vi "svx_Colormap Facade.vi"(0 "Data In":T5 {"Y scale"."multiplier" format="%.2f"; "Y scale"."offset" format="%.2f"; "X scale"."multiplier" format="%.2f"; "X scale"."offset" format="%.2f"; "spectral map" format="%.2f"}, 2 "Display State In":T3={"RefQueue"=refnum, "Properties/Undo"=refnum, "Bound"={"Width"=0, "Height"=0}, "Plot Area:Colors"={"FG Color"=11776947, "BG Color"=0}, "scale legend visible?"=FALSE, "graph palette visible?"=FALSE, "cursor palette visible?"=FALSE, "Ignore Array"=TRUE, "Smooth Update"=FALSE, "Z Scale"={"Z Scale.Scale Fit"=2, "Z Scale.Name Label.Text"="Amplitude", "Z Scale.Interpolate Color"=TRUE, "Visible"=TRUE, "Label Visible"=TRUE, "format string"="%#.2g", "Z Scale.Range"={"Minimum"=0.0, "Maximum"=500.0}}, "X Scale"={"X Scale.Scale Fit"=2, "X Scale.Offset and Multiplier"={"Offset"=0.0, "Multiplier"=1.0}, "X Scale.Name Label.Text"="Time", "X Scale.Range"={"Minimum"=0.0, "Maximum"=10.0}, "Visible"=TRUE, "Label Visible"=TRUE, "format string"="%#.2g"}, "Y Scale"={"Y Scale.Scale Fit"=2, "Y Scale.Offset and Multiplier"={"Offset"=0.0, "Multiplier"=1.0}, "Y Scale.Name Label.Text"="Frequency", "Y Scale.Range"={"Minimum"=0.0, "Maximum"=500.0}, "Visible"=TRUE, "Label Visible"=TRUE, "format string"="%#.2g"}, "Annotation List"=[], "Cursor List"=[], "Display Frequency Lines"=TRUE, "Display Order Lines"=TRUE, "Display Order text"=TRUE, "Display Frequency text"=TRUE, "Order Lineproperty"={"Line"={"Width"=1, "Style"=enum."Dash"}, "color"=0}, "Order Textproperty"={"Test size"=11, "color"=16777222, "background"=16777216}, "Orders"=[], "Frequency"=[], "Frequency Lineproperty"={"Line"={"Width"=1, "Style"=enum."Dash"}, "color"=0}, "Frequency Textproperty"={"Test size"=11, "color"=16777222, "background"=16777216}, "Display Order from Cursor"=FALSE, "Display Freq from Cursor"=FALSE, "Active Cursor"=0, "Selected Cursors"=[], "Cursor Move"=refnum, "Scale Range Change"=refnum}, 3 "Container State":T4) -> (6 "Data Out":T5 {"Y scale"."multiplier" format="%.2f"; "Y scale"."offset" format="%.2f"; "X scale"."multiplier" format="%.2f"; "X scale"."offset" format="%.2f"; "spectral map" format="%.2f"}, 7 "Display State Out":T3={"RefQueue"=refnum, "Properties/Undo"=refnum, "Bound"={"Width"=0, "Height"=0}, "Plot Area:Colors"={"FG Color"=11776947, "BG Color"=0}, "scale legend visible?"=FALSE, "graph palette visible?"=FALSE, "cursor palette visible?"=FALSE, "Ignore Array"=TRUE, "Smooth Update"=FALSE, "Z Scale"={"Z Scale.Scale Fit"=2, "Z Scale.Name Label.Text"="Amplitude", "Z Scale.Interpolate Color"=TRUE, "Visible"=TRUE, "Label Visible"=TRUE, "format string"="%#.2g", "Z Scale.Range"={"Minimum"=0.0, "Maximum"=500.0}}, "X Scale"={"X Scale.Scale Fit"=2, "X Scale.Offset and Multiplier"={"Offset"=0.0, "Multiplier"=1.0}, "X Scale.Name Label.Text"="Time", "X Scale.Range"={"Minimum"=0.0, "Maximum"=10.0}, "Visible"=TRUE, "Label Visible"=TRUE, "format string"="%#.2g"}, "Y Scale"={"Y Scale.Scale Fit"=2, "Y Scale.Offset and Multiplier"={"Offset"=0.0, "Multiplier"=1.0}, "Y Scale.Name Label.Text"="Frequency", "Y Scale.Range"={"Minimum"=0.0, "Maximum"=500.0}, "Visible"=TRUE, "Label Visible"=TRUE, "format string"="%#.2g"}, "Annotation List"=[], "Cursor List"=[], "Display Frequency Lines"=TRUE, "Display Order Lines"=TRUE, "Display Order text"=TRUE, "Display Frequency text"=TRUE, "Order Lineproperty"={"Line"={"Width"=1, "Style"=enum."Dash"}, "color"=0}, "Order Textproperty"={"Test size"=11, "color"=16777222, "background"=16777216}, "Orders"=[], "Frequency"=[], "Frequency Lineproperty"={"Line"={"Width"=1, "Style"=enum."Dash"}, "color"=0}, "Frequency Textproperty"={"Test size"=11, "color"=16777222, "background"=16777216}, "Display Order from Cursor"=FALSE, "Display Freq from Cursor"=FALSE, "Active Cursor"=0, "Selected Cursors"=[], "Cursor Move"=refnum, "Scale Range Change"=refnum}, 8 "Action":T2)   [LabVIEW 2017, in "SVX Colormap.xctl"]
uses:
  <vilib>/addons/_XControls/Colormap/SVX Colormap.xctl
  <vilib>/addons/_XControls/Colormap/subVIs/svx_Colormap Data.ctl
  <vilib>/_xctls/Container State.ctl
  <vilib>/addons/_XControls/Colormap/subVIs/svx_Colormap State.ctl
  <vilib>/addons/_XControls/Colormap/TypeDef/svx_Colormap_InnerState.ctl
  <vilib>/addons/_XControls/Colormap/TypeDef/svx_Colormap_Event.ctl
  <vilib>/_xctls/Action.ctl
  <vilib>/Utility/miscctls.llb/LVPoint32TypeDef.ctl
  <vilib>/_xctls/XControlSupport.lvlib
panel:
  in  "by cursor legend?":bool=TRUE
  out "Coords":T1
  out "Colormap":dbl[][](graph)
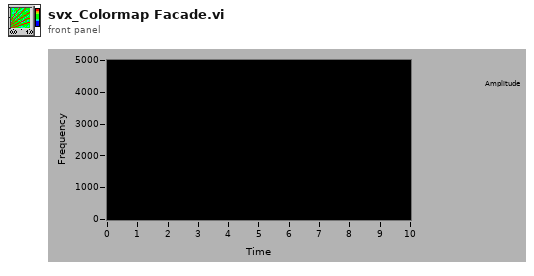
[diagram p1: front panel]
types:
  T1 = typedef "LVPoint32TypeDef.ctl" = cluster{"Horizontal":i32, "Vertical":i32}
  T2 = typedef "XControlSupport.lvlib/Action.ctl" = cluster{"Data Changed?":bool, "State Changed?":bool, "Action Name":string}
  T3 = typedef "SVX Colormap.xctl/svx_Colormap State.ctl" = cluster{"RefQueue":refnum<queue>, "Properties/Undo":refnum<queue>, "Bound":cluster{"Width":u32, "Height":u32}, "Plot Area:Colors":cluster{"FG Color":u32, "BG Color":u32}, "scale legend visible?":bool, "graph palette visible?":bool, "cursor palette visible?":bool, "Ignore Array":bool, "Smooth Update":bool, "Z Scale":cluster{"Z Scale.Scale Fit":u8, "Z Scale.Name Label.Text":string, "Z Scale.Interpolate Color":bool, "Visible":bool, "Label Visible":bool, "format string":string, "Z Scale.Range":cluster{"Minimum":dbl, "Maximum":dbl}}, "X Scale":cluster{"X Scale.Scale Fit":u8, "X Scale.Offset and Multiplier":cluster{"Offset":dbl, "Multiplier":dbl}, "X Scale.Name Label.Text":string, "X Scale.Range":cluster{"Minimum":dbl, "Maximum":dbl}, "Visible":bool, "Label Visible":bool, "format string":string}, "Y Scale":cluster{"Y Scale.Scale Fit":u8, "Y Scale.Offset and Multiplier":cluster{"Offset":dbl, "Multiplier":dbl}, "Y Scale.Name Label.Text":string, "Y Scale.Range":cluster{"Minimum":dbl, "Maximum":dbl}, "Visible":bool, "Label Visible":bool, "format string":string}, "Annotation List":cluster{"Name":string, "Color":u32, "Style":u8, "Point Style":u8, "Name Visible":bool, "Allow Drag":bool, "Annotation Mode":u32, "Plot":i32, "Index":i32, "Position":cluster{"X":dbl, "Y":dbl}, "X Scale":u32, "Y Scale":u32, "Show Arrow":bool, "Lock Name":bool, "Plot Area":i32, "Label Offset":cluster{"X":dbl, "Y":dbl}}[], "Cursor List":cluster{"Name":string, "Color":u32, "Style":u8, "Point Style":u8, "Name Visible":bool, "Allow Drag":bool, "Cursor Mode":u32, "Plot":i32, "Index":i32, "Position":cluster{"X":dbl, "Y":dbl}, "X Scale":u32, "Y Scale":u32, "Watch Plots":i32[], "Watch All Plots":bool, "Plot Area":i32, "Label Offset":cluster{"X":dbl, "Y":dbl}}[], "Display Frequency Lines":bool, "Display Order Lines":bool, "Display Order text":bool, "Display Frequency text":bool, "Order Lineproperty":cluster{"Line":cluster{"Width":u16, "Style":enum32{"Solid", "Dash", "Dot", "DashDot", "DashDotDot"}}, "color":u32}, "Order Textproperty":cluster{"Test size":i16, "color":u32, "background":u32}, "Orders":dbl[], "Frequency":dbl[], "Frequency Lineproperty":cluster{"Line":cluster{"Width":u16, "Style":enum32{"Solid", "Dash", "Dot", "DashDot", "DashDotDot"}}, "color":u32}, "Frequency Textproperty":cluster{"Test size":i16, "color":u32, "background":u32}, "Display Order from Cursor":bool, "Display Freq from Cursor":bool, "Active Cursor":u32, "Selected Cursors":u32[], "Cursor Move":refnum<user-event>, "Scale Range Change":refnum<user-event>}
  T4 = typedef "XControlSupport.lvlib/Container State.ctl" = cluster{"Indicator?":bool, "Run Mode?":bool, " Refnum":refnum<vi>}
  T5 = typedef "SVX Colormap.xctl/svx_Colormap Data.ctl" = cluster{"spectral map":dbl[][], "X scale":cluster{"offset":dbl, "multiplier":dbl}, "Y scale":cluster{"offset":dbl, "multiplier":dbl}, "attribute":variant}
  T6 = cluster{"Minimum":dbl, "Maximum":dbl, "Kind":enum16{"X-Scale", "Y-Scale", "Z-Scale"}}
  T7 = typedef "SVX Colormap.xctl/svx_Colormap_Event.ctl" = enum16{"None", "[Axis] X Range", "[Axis] Y Range", "[Axis] Z Range", "[Axis] Range", "[Axis] X FString", "[Axis] Y FString", "[Axis] Z FString", "[Axis] X Name", "[Axis] X ScaleVis", "[Axis] X NameVis", "[Axis] Y Name", "[Axis] Y ScaleVis", "[Axis] Y NameVis", "[Axis] Z Name", "[Axis] Z ScaleVis", "[Axis] Z NameVis", "[Image] Line", "[Axis] Z Interp", "[Data] Update", "[Layout] Resize", "[ColorTable] Ignore Array", "[Legend] ScaleVis", "[Legend] GPVis", "[Legend] CPVis", "[Smooth] Update", "[Cursor] Update", "[Plot Area] Colors", "[Size] Minimum", "[Annotation] Update", "[Properties Dialog]", "[Axis] Autoscale X", "[Axis] Autoscale Y", "[Axis] Autoscale Z"}
  T8 = typedef "LVRectTypeDef.ctl" = cluster{"Left":i16, "Top":i16, "Right":i16, "Bottom":i16}
  T9 = typedef "LVCursorListTypeDef.ctl" = cluster{"Name":string, "Color":u32, "Style":u8, "Point Style":u8, "Name Visible":bool, "Allow Drag":bool, "Cursor Mode":u32, "Plot":i32, "Index":i32, "Position":cluster{"X":dbl, "Y":dbl}, "X Scale":u32, "Y Scale":u32, "Watch Plots":i32[], "Watch All Plots":bool, "Plot Area":i32, "Label Offset":cluster{"X":dbl, "Y":dbl}}[]
  T10 = cluster{"Shift":bool, "Ctrl":bool, "Alt":bool, "Cmd":bool, "Opt":bool}
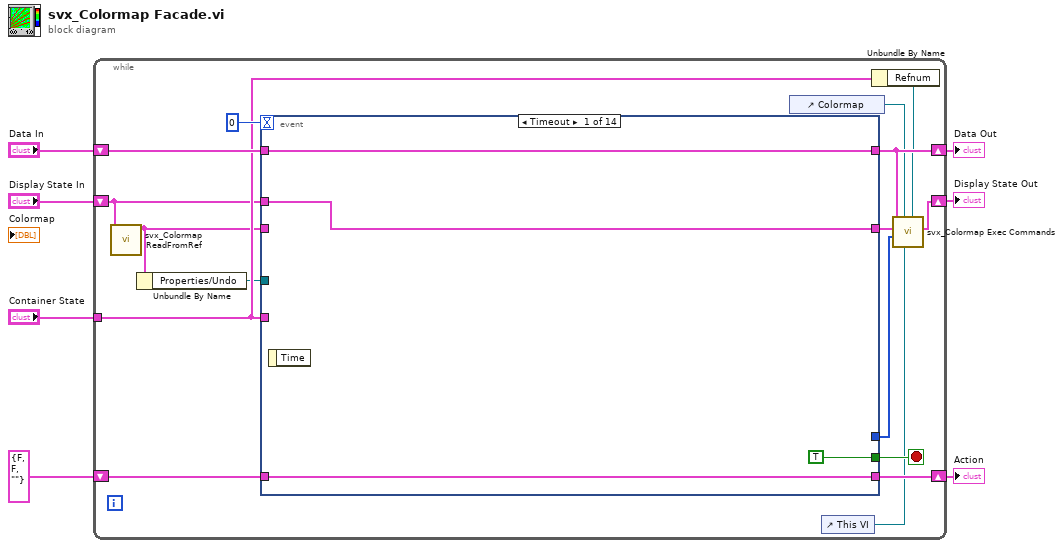
[diagram p0: block diagram]
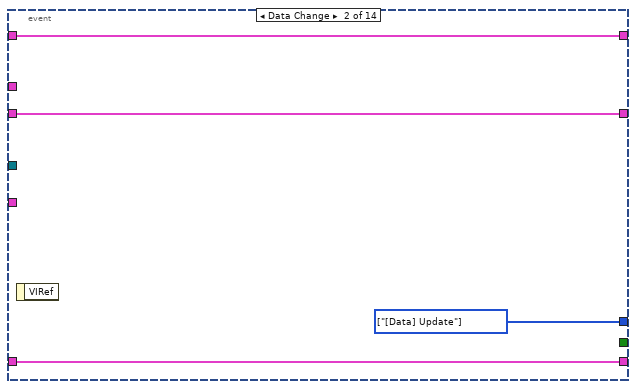
[diagram p2: hidden frame]
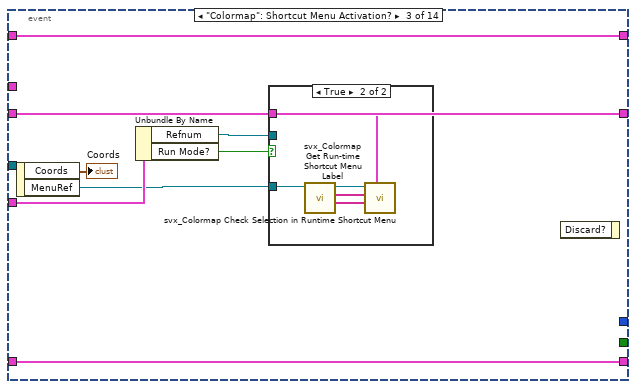
[diagram p3: hidden frame]
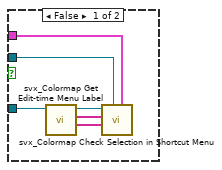
[diagram p4: hidden frame]
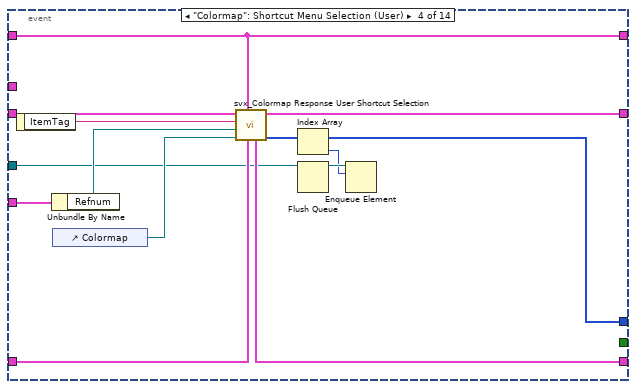
[diagram p5: hidden frame]
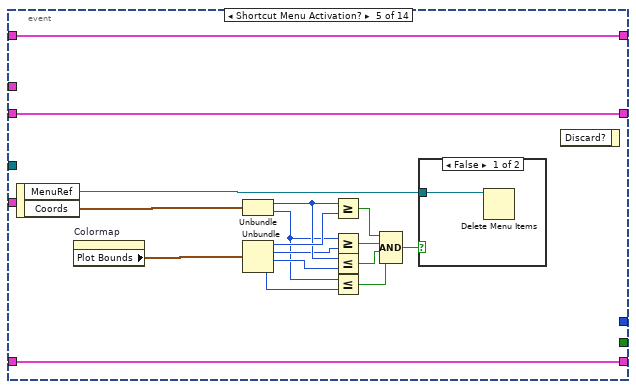
[diagram p6: hidden frame]
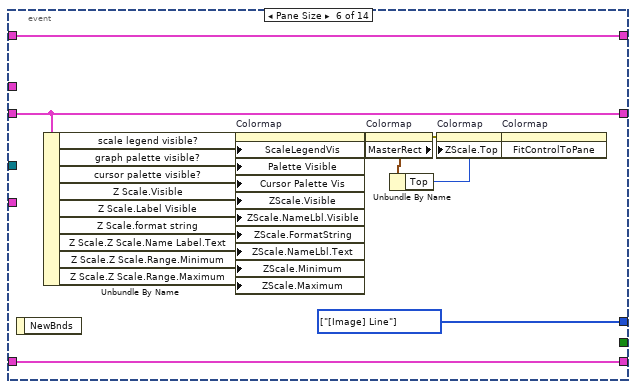
[diagram p8: hidden frame]
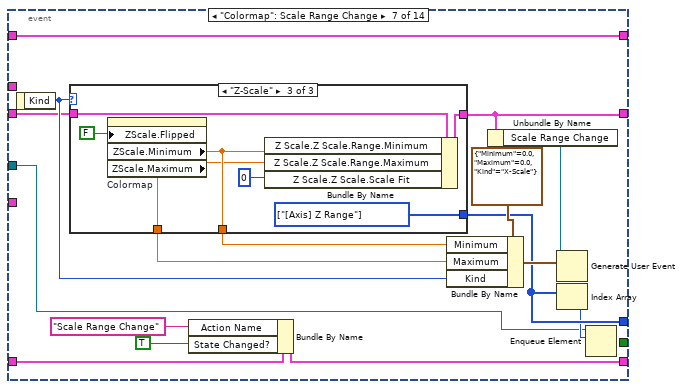
[diagram p9: hidden frame]
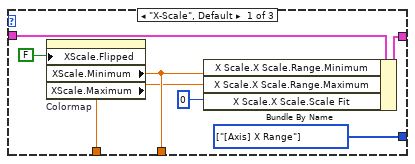
[diagram p10: hidden frame]
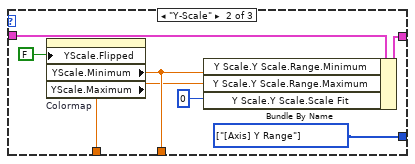
[diagram p11: hidden frame]
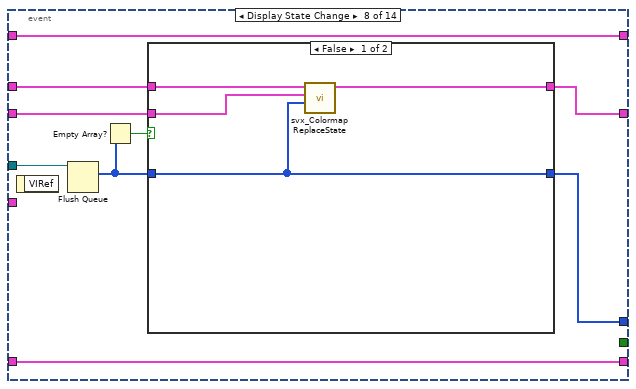
[diagram p12: hidden frame]
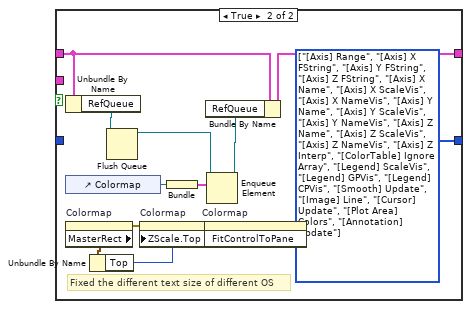
[diagram p13: hidden frame]
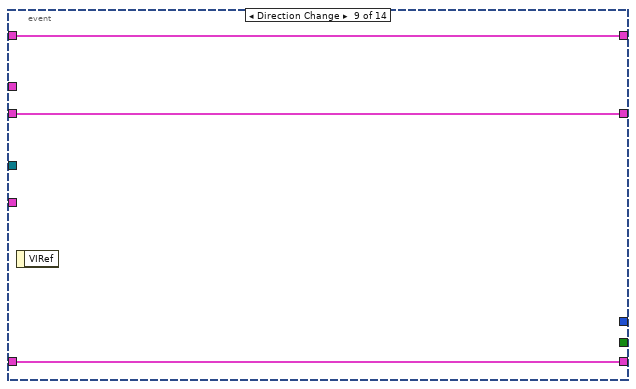
[diagram p14: hidden frame]
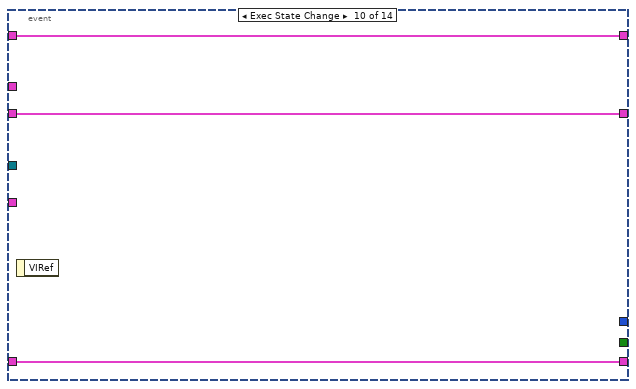
[diagram p15: hidden frame]
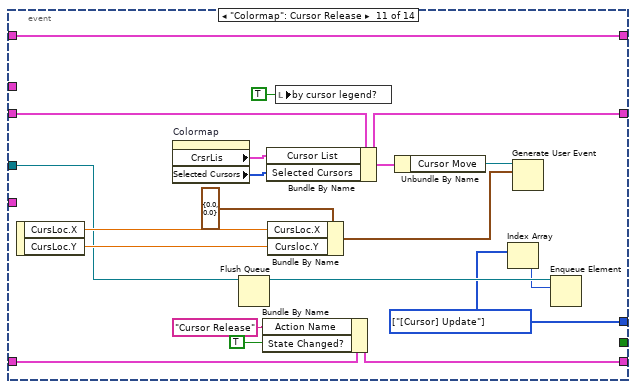
[diagram p16: hidden frame]
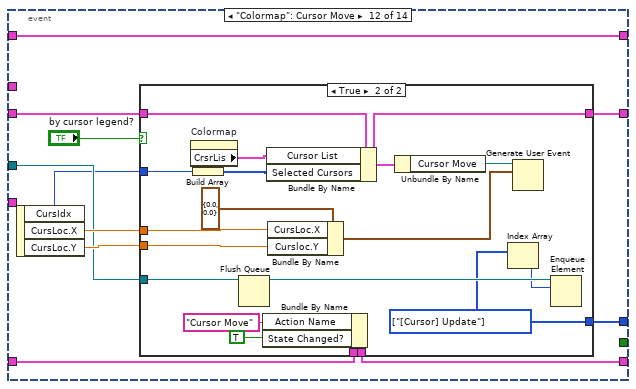
[diagram p17: hidden frame]
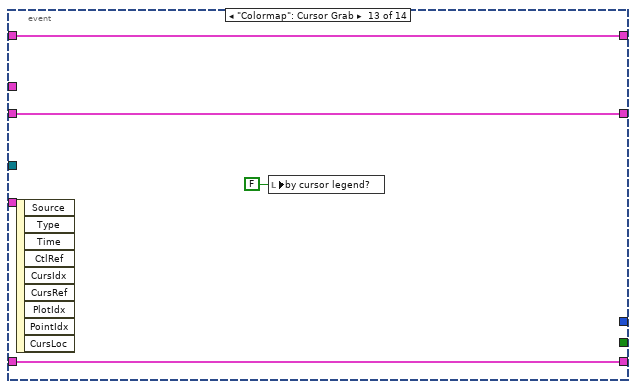
[diagram p19: hidden frame]
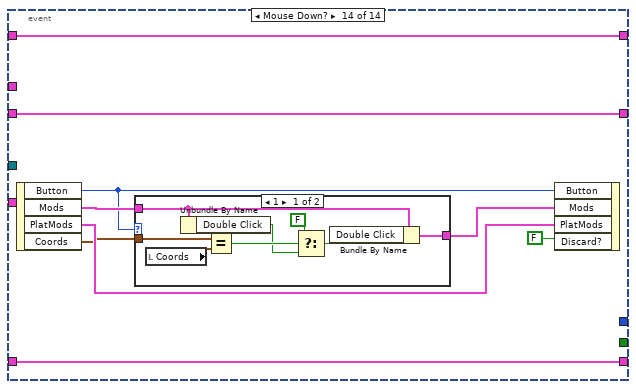
[diagram p20: hidden frame]
diagram:
  n1 = while {
    shift-right: [w8] -> w4
    shift-left: "Display State In" -> [w10]
    tunnel: "Container State" -> [w19]
    shift-right: [w20] -> w2
    shift-left: "Data In" -> [w22]
    shift-right: [w15] -> w3
    shift-left: T2 {"Data Changed?"=FALSE, "State Changed?"=FALSE, "Action Name"=""} ("Action") -> [w21]
    stop <- w13 stop-if-true
    n2 = call <vilib>:"svx_Colormap ReadFromRef.vi"("State in"=w10) -> ("State out"=w11:T3)  [unwired: 10 in]
    n3 = Unbundle By Name(w11) -> ("Properties/Undo"=w14:refnum<queue>)
    n4 = event shown="[0] Timeout" {
      selector: _ -> [_ _ _ _ _ _ _ _ _ _ _ _ _ _]
      dyn-events: _ -> [_ _ _ _ _ _ _ _ _ _ _ _ _ _]
      timeout: 0 -> [_ _ _ _ _ _ _ _ _ _ _ _ _ _]
      tunnel: w19 -> [_ _ w36 w61 _ _ _ _ _ _ _ _ _ _]
      tunnel: w22 -> [w27 w31 w39 w60 w79 w98 w111 w145 w164 w167 w183 w195 w219 w230]
      tunnel: [w27 w31 w39 w60 w79 w98 w111 w145 w164 w167 w183 w195 w219 w230] -> w20
      tunnel: [w26 w30 w38 w62 w80 w99 w113 w144 w163 w166 w184 w196 w218 w228] -> w15
      tunnel: w21 -> [w26 w30 w38 w63 w80 w99 w114 w144 w163 w166 w185 w197 w218 w228]
      tunnel: w10 -> [w24 _ _ _ _ _ _ w139 _ _ _ _ _ _]
      tunnel: w14 -> [_ _ _ w52 _ _ w100 w143 _ _ w172 w190 _ _]
      tunnel: [_ w29 _ w51 _ w97 w102 w140 _ _ w170 w189 _ _] -> w16
      tunnel: w11 -> [_ w28 w33 w59 w64 w82 w105 w137 w162 w165 w177 w192 w220 w229]
      tunnel: [w24 w28 w33 w58 w64 w82 w104 w138 w162 w165 w175 w191 w220 w229] -> w9
      tunnel: [TRUE _ _ _ _ _ _ _ _ _ _ _ _ _] -> w13
      event Timeout {
        n5 = event-data() -> ()  [unwired: 1 in, 1 out]
      }
      event Data Change {
        w29 = T7[] [enum."[Data] Update"] items=["None", "[Axis] X Range", "[Axis] Y Range", "[Axis] Z Range", "[Axis] Range", "[Axis] X FString", "[Axis] Y FString", "[Axis] Z FString", "[Axis] X Name", "[Axis] X ScaleVis", "[Axis] X NameVis", "[Axis] Y Name", "[Axis] Y ScaleVis", "[Axis] Y NameVis", "[Axis] Z Name", "[Axis] Z ScaleVis", "[Axis] Z NameVis", "[Image] Line", "[Axis] Z Interp", "[Data] Update", "[Layout] Resize", "[ColorTable] Ignore Array", "[Legend] ScaleVis", "[Legend] GPVis", "[Legend] CPVis", "[Smooth] Update", "[Cursor] Update", "[Plot Area] Colors", "[Size] Minimum", "[Annotation] Update", "[Properties Dialog]", "[Axis] Autoscale X", "[Axis] Autoscale Y", "[Axis] Autoscale Z"]
        n6 = event-data() -> ()  [unwired: 1 in, 1 out]
      }
      event "Colormap": Shortcut Menu Activation? {
        n7 = event-data() -> ("Coords"=→"Coords":T1, "MenuRef"=w34:refnum<k9>)  [unwired: 1 in]
        n8 = Unbundle By Name(w36) -> ("Refnum"=w35:refnum<vi>, "Run Mode?"=w37:bool)
        n9 = case shown="True" w37 {
          tunnel: w34 -> [w45 w50]
          tunnel: w35 -> [w42 _]
          tunnel: w33 -> [w41 w46]
          frame False {
            n10 = call <vilib>:"svx_Colormap Get Edit-time Menu Label.vi"("MenuRef"=w45) -> ("Disable item tags"=w40:string[], "item tags"=w43:string[], "menu reference out"=w44:refnum<k9>)  [unwired: 8 in]
            n11 = call <vilib>:"svx_Colormap Check Selection in Shortcut Menu.vi"("State"=w41, "Refnum"=w42, "Disable item tags"=w40, "item tags"=w43, "menu reference in"=w44) -> ()  [unwired: 7 in]
          }
          frame True {
            n12 = call <vilib>:"svx_Colormap Get Run-time Shortcut Menu Label.vi"("MenuRef"=w50) -> ("Disable item tags"=w47:string[], "item tags"=w48:string[], "menu reference out"=w49:refnum<k9>)  [unwired: 8 in]
            n13 = call <vilib>:"svx_Colormap Check Selection in Runtime Shortcut Menu.vi"("State"=w46, "Disable item tags"=w47, "item tags"=w48, "menu reference in"=w49) -> ()  [unwired: 8 in]
          }
        }
        n14 = event-data() -> ()  [unwired: 2 in, 1 out]
      }
      event "Colormap": Shortcut Menu Selection (User) {
        n15 = event-data() -> ("ItemTag"=w57:string)  [unwired: 1 in]
        n16 = Unbundle By Name(w61) -> ("Refnum"=w56:refnum<vi>)
        n17 = control-ref of="Colormap"() -> (w55:refnum<vi>)
        n18 = call <vilib>:"svx_Colormap Response User Shortcut Selection.vi"("Action In"=w63, "Data In"=w60, "Color Map in"=w55, "Refnum"=w56, "ItemTag"=w57, "State in"=w59) -> ("Events"=w51:T7[], "State out"=w58:T3, "Action"=w62:T2)  [unwired: 3 in]
        n19 = Index Array(array=w51) -> (element=w53:T7)  [unwired: 1 in]
        n20 = Flush Queue(queue=w52) -> (queue out=w54:refnum<queue>)  [unwired: 1 in, 2 out]
        n21 = Enqueue Element(queue=w54, element=w53) -> ()  [unwired: 2 in, 3 out]
      }
      event Shortcut Menu Activation? {
        n22 = event-data() -> ("MenuRef"=w66:refnum<k9>, "Coords"=w78:T1)  [unwired: 1 in]
        n23 = property on="Colormap" class="IntGraph (strict)"() -> ("Plot Bounds"=w65:T8)  [unwired: 2 in, 2 out]
        n24 = Unbundle(w78) -> ("Horizontal"=w76:i32, "Vertical"=w73:i32)
        n25 = Unbundle(w65) -> ("Left"=w77:i16, "Top"=w74:i16, "Right"=w75:i16, "Bottom"=w72:i16)
        n26 = Greater Or Equal?(x=w76, y=w77) -> (x >= y?=w71:bool)
        n27 = Greater Or Equal?(x=w73, y=w74) -> (x >= y?=w70:bool)
        n28 = Less Or Equal?(x=w76, y=w75) -> (x <= y?=w69:bool)
        n29 = Less Or Equal?(x=w73, y=w72) -> (x <= y?=w68:bool)
        n30 = Compound Arithmetic op=AND(w71, w70, w69, w68) -> (w67:bool)
        n31 = case shown="False" w67 {
          tunnel: w66 -> [w81 _]
          frame False {
            n32 = Delete Menu Items(9:w81) -> ()  [unwired: 3 in, 2 out]
          }
          frame True {
          }
        }
        n33 = event-data() -> ()  [unwired: 2 in, 1 out]
      }
      event Pane Size {
        w97 = T7[] [enum."[Image] Line"] items=["None", "[Axis] X Range", "[Axis] Y Range", "[Axis] Z Range", "[Axis] Range", "[Axis] X FString", "[Axis] Y FString", "[Axis] Z FString", "[Axis] X Name", "[Axis] X ScaleVis", "[Axis] X NameVis", "[Axis] Y Name", "[Axis] Y ScaleVis", "[Axis] Y NameVis", "[Axis] Z Name", "[Axis] Z ScaleVis", "[Axis] Z NameVis", "[Image] Line", "[Axis] Z Interp", "[Data] Update", "[Layout] Resize", "[ColorTable] Ignore Array", "[Legend] ScaleVis", "[Legend] GPVis", "[Legend] CPVis", "[Smooth] Update", "[Cursor] Update", "[Plot Area] Colors", "[Size] Minimum", "[Annotation] Update", "[Properties Dialog]", "[Axis] Autoscale X", "[Axis] Autoscale Y", "[Axis] Autoscale Z"] ("Events")
        n34 = event-data() -> ()  [unwired: 1 in, 1 out]
        n35 = Unbundle By Name(w82) -> ("scale legend visible?"=w91:bool, "graph palette visible?"=w90:bool, "cursor palette visible?"=w89:bool, "Z Scale.Visible"=w88:bool, "Z Scale.Label Visible"=w87:bool, "Z Scale.format string"=w86:string, "Z Scale.Z Scale.Name Label.Text"=w85:string, "Z Scale.Z Scale.Range.Minimum"=w84:dbl, "Z Scale.Z Scale.Range.Maximum"=w83:dbl)
        n36 = property on="Colormap" class="IntGraph (strict)"("ScaleLegendVis"=w91, "Palette Visible"=w90, "Cursor Palette Vis"=w89, "ZScale.Visible"=w88, "ZScale.NameLbl.Visible"=w87, "ZScale.FormatString"=w86, "ZScale.NameLbl.Text"=w85, "ZScale.Minimum"=w84, "ZScale.Maximum"=w83) -> (error out=w93:errorcluster)  [unwired: 2 in, 1 out]
        n37 = property on="Colormap" class="IntGraph (strict)"(error in=w93) -> (error out=w94:errorcluster, "MasterRect"=w95:T8)  [unwired: 1 in, 1 out]
        n38 = Unbundle By Name(w95) -> ("Top"=w96:i16)
        n39 = property on="Colormap" class="IntGraph (strict)"(error in=w94, "ZScale.Top"=w96) -> (error out=w92:errorcluster)  [unwired: 1 in, 1 out]
        n40 = invoke on="Colormap" class="IntGraph (strict)" method="FitControlToPane"(error in=w92) -> ()  [unwired: 2 in, 3 out]
      }
      event "Colormap": Scale Range Change {
        n41 = event-data() -> ("Kind"=w108:enum16{"X-Scale", "Y-Scale", "Z-Scale"})  [unwired: 1 in]
        n42 = case shown="\"Z-Scale\"" w108 {
          tunnel: [w122 w129 w136] -> w110
          tunnel: [w121 w128 w135] -> w109
          tunnel: w105 -> [w118 w125 w132]
          tunnel: [w117 w124 w131] -> w104
          tunnel: [w116 w123 w130] -> w102
          frame "X-Scale", Default {
            w116 = T7[] [enum."[Axis] X Range"] items=["None", "[Axis] X Range", "[Axis] Y Range", "[Axis] Z Range", "[Axis] Range", "[Axis] X FString", "[Axis] Y FString", "[Axis] Z FString", "[Axis] X Name", "[Axis] X ScaleVis", "[Axis] X NameVis", "[Axis] Y Name", "[Axis] Y ScaleVis", "[Axis] Y NameVis", "[Axis] Z Name", "[Axis] Z ScaleVis", "[Axis] Z NameVis", "[Image] Line", "[Axis] Z Interp", "[Data] Update", "[Layout] Resize", "[ColorTable] Ignore Array", "[Legend] ScaleVis", "[Legend] GPVis", "[Legend] CPVis", "[Smooth] Update", "[Cursor] Update", "[Plot Area] Colors", "[Size] Minimum", "[Annotation] Update", "[Properties Dialog]", "[Axis] Autoscale X", "[Axis] Autoscale Y", "[Axis] Autoscale Z"] ("Events")
            n43 = property on="Colormap" class="IntGraph (strict)"("XScale.Flipped"=FALSE ("X Scale.Flipped")) -> ("XScale.Minimum"=w122:dbl, "XScale.Maximum"=w121:dbl)  [unwired: 2 in, 2 out]
            n44 = Bundle By Name(cluster=w118, "X Scale.X Scale.Range.Minimum"=w122, "X Scale.X Scale.Range.Maximum"=w121, "X Scale.X Scale.Scale Fit"=u8 0 ("X Scale.Scale Fit")) -> (w117:T3)
          }
          frame "Y-Scale" {
            w123 = T7[] [enum."[Axis] Y Range"] items=["None", "[Axis] X Range", "[Axis] Y Range", "[Axis] Z Range", "[Axis] Range", "[Axis] X FString", "[Axis] Y FString", "[Axis] Z FString", "[Axis] X Name", "[Axis] X ScaleVis", "[Axis] X NameVis", "[Axis] Y Name", "[Axis] Y ScaleVis", "[Axis] Y NameVis", "[Axis] Z Name", "[Axis] Z ScaleVis", "[Axis] Z NameVis", "[Image] Line", "[Axis] Z Interp", "[Data] Update", "[Layout] Resize", "[ColorTable] Ignore Array", "[Legend] ScaleVis", "[Legend] GPVis", "[Legend] CPVis", "[Smooth] Update", "[Cursor] Update", "[Plot Area] Colors", "[Size] Minimum", "[Annotation] Update", "[Properties Dialog]", "[Axis] Autoscale X", "[Axis] Autoscale Y", "[Axis] Autoscale Z"] ("Events")
            n45 = property on="Colormap" class="IntGraph (strict)"("YScale.Flipped"=FALSE ("X Scale.Flipped")) -> ("YScale.Minimum"=w129:dbl, "YScale.Maximum"=w128:dbl)  [unwired: 2 in, 2 out]
            n46 = Bundle By Name(cluster=w125, "Y Scale.Y Scale.Range.Minimum"=w129, "Y Scale.Y Scale.Range.Maximum"=w128, "Y Scale.Y Scale.Scale Fit"=u8 0 ("X Scale.Scale Fit")) -> (w124:T3)
          }
          frame "Z-Scale" {
            w130 = T7[] [enum."[Axis] Z Range"] items=["None", "[Axis] X Range", "[Axis] Y Range", "[Axis] Z Range", "[Axis] Range", "[Axis] X FString", "[Axis] Y FString", "[Axis] Z FString", "[Axis] X Name", "[Axis] X ScaleVis", "[Axis] X NameVis", "[Axis] Y Name", "[Axis] Y ScaleVis", "[Axis] Y NameVis", "[Axis] Z Name", "[Axis] Z ScaleVis", "[Axis] Z NameVis", "[Image] Line", "[Axis] Z Interp", "[Data] Update", "[Layout] Resize", "[ColorTable] Ignore Array", "[Legend] ScaleVis", "[Legend] GPVis", "[Legend] CPVis", "[Smooth] Update", "[Cursor] Update", "[Plot Area] Colors", "[Size] Minimum", "[Annotation] Update", "[Properties Dialog]", "[Axis] Autoscale X", "[Axis] Autoscale Y", "[Axis] Autoscale Z"] ("Events")
            n47 = property on="Colormap" class="IntGraph (strict)"("ZScale.Flipped"=FALSE ("X Scale.Flipped")) -> ("ZScale.Minimum"=w136:dbl, "ZScale.Maximum"=w135:dbl)  [unwired: 2 in, 2 out]
            n48 = Bundle By Name(cluster=w132, "Z Scale.Z Scale.Range.Minimum"=w136, "Z Scale.Z Scale.Range.Maximum"=w135, "Z Scale.Z Scale.Scale Fit"=u8 0 ("X Scale.Scale Fit")) -> (w131:T3)
          }
        }
        n49 = Bundle By Name(cluster=w114, "Action Name"="Scale Range Change", "State Changed?"=TRUE) -> (w113:T2)
        n50 = Bundle By Name(cluster=T6 {"Minimum"=0.0, "Maximum"=0.0, "Kind"=enum."X-Scale"} ("output cluster"), "Minimum"=w110, "Maximum"=w109, "Kind"=w108) -> (w106:T6)
        n51 = Unbundle By Name(w104) -> ("Scale Range Change"=w103:refnum<user-event>)
        n52 = Generate User Event(user event=w103, event data cluster=w106) -> ()  [unwired: 2 in, 2 out]
        n53 = Index Array(array=w102) -> (element=w101:T7)  [unwired: 1 in]
        n54 = Enqueue Element(queue=w100, element=w101) -> ()  [unwired: 2 in, 3 out]
      }
      event Display State Change {
        n55 = event-data() -> ()  [unwired: 1 in, 1 out]
        n56 = Flush Queue(queue=w143) -> (remaining elements=w141:T7[])  [unwired: 1 in, 2 out]
        n57 = Empty Array?(array=w141) -> (empty?=w142:bool)
        n58 = case shown="False" w142 {
          tunnel: w141 -> [w149 _]
          tunnel: [w149 w161] -> w140
          tunnel: w139 -> [w147 w155]
          tunnel: [w146 w154] -> w138
          tunnel: w137 -> [w148 _]
          frame False {
            n59 = call <vilib>:"svx_Colormap ReplaceState.vi"("Events"=w149, "RefState"=w148, "NewState"=w147) -> ("State out"=w146:T3)  [unwired: 8 in]
          }
          frame True {
            w161 = T7[] [enum."[Axis] Range", enum."[Axis] X FString", enum."[Axis] Y FString", enum."[Axis] Z FString", enum."[Axis] X Name", enum."[Axis] X ScaleVis", enum."[Axis] X NameVis", enum."[Axis] Y Name", enum."[Axis] Y ScaleVis", enum."[Axis] Y NameVis", enum."[Axis] Z Name", enum."[Axis] Z ScaleVis", enum."[Axis] Z NameVis", enum."[Axis] Z Interp", enum."[ColorTable] Ignore Array", enum."[Legend] ScaleVis", enum."[Legend] GPVis", enum."[Legend] CPVis", enum."[Smooth] Update", enum."[Image] Line", enum."[Cursor] Update", enum."[Plot Area] Colors", enum."[Annotation] Update"] items=["None", "[Axis] X Range", "[Axis] Y Range", "[Axis] Z Range", "[Axis] Range", "[Axis] X FString", "[Axis] Y FString", "[Axis] Z FString", "[Axis] X Name", "[Axis] X ScaleVis", "[Axis] X NameVis", "[Axis] Y Name", "[Axis] Y ScaleVis", "[Axis] Y NameVis", "[Axis] Z Name", "[Axis] Z ScaleVis", "[Axis] Z NameVis", "[Image] Line", "[Axis] Z Interp", "[Data] Update", "[Layout] Resize", "[ColorTable] Ignore Array", "[Legend] ScaleVis", "[Legend] GPVis", "[Legend] CPVis", "[Smooth] Update", "[Cursor] Update", "[Plot Area] Colors", "[Size] Minimum", "[Annotation] Update", "[Properties Dialog]", "[Axis] Autoscale X", "[Axis] Autoscale Y", "[Axis] Autoscale Z"] ("remaining elements")
            # "Fixed the different text size of different OS"
            n60 = Unbundle By Name(w155) -> ("RefQueue"=w160:refnum<queue>)
            n61 = control-ref of="Colormap"() -> (w159:refnum<vi>)
            n62 = property on="Colormap" class="IntGraph (strict)"() -> (error out=w152:errorcluster, "MasterRect"=w151:T8)  [unwired: 2 in, 1 out]
            n63 = Unbundle By Name(w151) -> ("Top"=w150:i16)
            n64 = Flush Queue(queue=w160) -> (queue out=w157:refnum<queue>)  [unwired: 1 in, 2 out]
            n65 = property on="Colormap" class="IntGraph (strict)"(error in=w152, "ZScale.Top"=w150) -> (error out=w153:errorcluster)  [unwired: 1 in, 1 out]
            n66 = Bundle("Colormap"=w159) -> (w158:cluster{"Colormap":refnum<vi>})  [unwired: 1 in]
            n67 = invoke on="Colormap" class="IntGraph (strict)" method="FitControlToPane"(error in=w153) -> ()  [unwired: 2 in, 3 out]
            n68 = Enqueue Element(queue=w157, element=w158) -> (queue out=w156:refnum<queue>)  [unwired: 2 in, 2 out]
            n69 = Bundle By Name(cluster=w155, "RefQueue"=w156) -> (w154:T3)
          }
        }
      }
      event Direction Change {
        n70 = event-data() -> ()  [unwired: 1 in, 1 out]
      }
      event Exec State Change {
        n71 = event-data() -> ()  [unwired: 1 in, 1 out]
      }
      event "Colormap": Cursor Release {
        w170 = T7[] [enum."[Cursor] Update"] items=["None", "[Axis] X Range", "[Axis] Y Range", "[Axis] Z Range", "[Axis] Range", "[Axis] X FString", "[Axis] Y FString", "[Axis] Z FString", "[Axis] X Name", "[Axis] X ScaleVis", "[Axis] X NameVis", "[Axis] Y Name", "[Axis] Y ScaleVis", "[Axis] Y NameVis", "[Axis] Z Name", "[Axis] Z ScaleVis", "[Axis] Z NameVis", "[Image] Line", "[Axis] Z Interp", "[Data] Update", "[Layout] Resize", "[ColorTable] Ignore Array", "[Legend] ScaleVis", "[Legend] GPVis", "[Legend] CPVis", "[Smooth] Update", "[Cursor] Update", "[Plot Area] Colors", "[Size] Minimum", "[Annotation] Update", "[Properties Dialog]", "[Axis] Autoscale X", "[Axis] Autoscale Y", "[Axis] Autoscale Z"] ("Events")
        n72 = event-data() -> ("CursLoc.X"=w180:dbl, "CursLoc.Y"=w179:dbl)  [unwired: 1 in]
        n73 = property on="Colormap" class="IntGraph (strict)"() -> ("CrsrLis"=w182:T9, "Selected Cursors"=w174:u32[])  [unwired: 2 in, 2 out]
        n74 = Flush Queue(queue=w172) -> (queue out=w171:refnum<queue>)  [unwired: 1 in, 2 out]
        n75 = Bundle By Name(cluster=w185, "Action Name"="Cursor Release", "State Changed?"=TRUE) -> (w184:T2)
        n76 = Bundle By Name(cluster=w177, "Cursor List"=w182, "Selected Cursors"=w174) -> (w175:T3)
        n77 = Bundle By Name(cluster=cluster{"CursLoc.X":dbl, "Cursloc.Y":dbl} {"CursLoc.X"=0.0, "Cursloc.Y"=0.0} ("CursLoc"), "CursLoc.X"=w180, "Cursloc.Y"=w179) -> (w178:cluster{"CursLoc.X":dbl, "Cursloc.Y":dbl})
        n78 = local write "by cursor legend?"(TRUE ("by cursor legend?")) -> ()
        n79 = Unbundle By Name(w175) -> ("Cursor Move"=w176:refnum<user-event>)
        n80 = Index Array(array=w170) -> (element=w169:T7)  [unwired: 1 in]
        n81 = Generate User Event(user event=w176, event data cluster=w178) -> ()  [unwired: 2 in, 2 out]
        n82 = Enqueue Element(queue=w171, element=w169) -> ()  [unwired: 2 in, 3 out]
      }
      event "Colormap": Cursor Move {
        n83 = event-data() -> ("CursIdx"=w187:i32, "CursLoc.X"=w194:dbl, "CursLoc.Y"=w193:dbl)  [unwired: 1 in]
        n84 = case shown="True" "by cursor legend?" {
          tunnel: w197 -> [w198 w216]
          tunnel: [w198 w215] -> w196
          tunnel: w194 -> [_ w212]
          tunnel: w193 -> [_ w211]
          tunnel: w192 -> [w199 w209]
          tunnel: [w199 w207] -> w191
          tunnel: w190 -> [_ w205]
          tunnel: [_ w203] -> w189
          tunnel: w187 -> [_ w200]
          frame False {
          }
          frame True {
            w203 = T7[] [enum."[Cursor] Update"] items=["None", "[Axis] X Range", "[Axis] Y Range", "[Axis] Z Range", "[Axis] Range", "[Axis] X FString", "[Axis] Y FString", "[Axis] Z FString", "[Axis] X Name", "[Axis] X ScaleVis", "[Axis] X NameVis", "[Axis] Y Name", "[Axis] Y ScaleVis", "[Axis] Y NameVis", "[Axis] Z Name", "[Axis] Z ScaleVis", "[Axis] Z NameVis", "[Image] Line", "[Axis] Z Interp", "[Data] Update", "[Layout] Resize", "[ColorTable] Ignore Array", "[Legend] ScaleVis", "[Legend] GPVis", "[Legend] CPVis", "[Smooth] Update", "[Cursor] Update", "[Plot Area] Colors", "[Size] Minimum", "[Annotation] Update", "[Properties Dialog]", "[Axis] Autoscale X", "[Axis] Autoscale Y", "[Axis] Autoscale Z"] ("Events")
            n85 = property on="Colormap" class="IntGraph (strict)"() -> ("CrsrLis"=w214:T9)  [unwired: 2 in, 2 out]
            n86 = Build Array(w200) -> (w201:i32[])
            n87 = Flush Queue(queue=w205) -> (queue out=w204:refnum<queue>)  [unwired: 1 in, 2 out]
            n88 = Bundle By Name(cluster=w216, "Action Name"="Cursor Move", "State Changed?"=TRUE) -> (w215:T2)
            n89 = Bundle By Name(cluster=w209, "Cursor List"=w214, "Selected Cursors"=w201) -> (w207:T3)
            n90 = Bundle By Name(cluster=cluster{"CursLoc.X":dbl, "Cursloc.Y":dbl} {"CursLoc.X"=0.0, "Cursloc.Y"=0.0} ("CursLoc"), "CursLoc.X"=w212, "Cursloc.Y"=w211) -> (w210:cluster{"CursLoc.X":dbl, "Cursloc.Y":dbl})
            n91 = Unbundle By Name(w207) -> ("Cursor Move"=w208:refnum<user-event>)
            n92 = Index Array(array=w203) -> (element=w202:T7)  [unwired: 1 in]
            n93 = Generate User Event(user event=w208, event data cluster=w210) -> ()  [unwired: 2 in, 2 out]
            n94 = Enqueue Element(queue=w204, element=w202) -> ()  [unwired: 2 in, 3 out]
          }
        }
      }
      event "Colormap": Cursor Grab {
        n95 = event-data() -> ()  [unwired: 1 in, 9 out]
        n96 = local write "by cursor legend?"(FALSE ("by cursor legend?")) -> ()
      }
      event Mouse Down? {
        n97 = event-data() -> ("Button"=w223:u16, "Mods"=w227:cluster{"Double Click":bool, "Menu Key":bool}, "PlatMods"=w225:T10, "Coords"=w222:T1)  [unwired: 1 in]
        n98 = case shown="1" w223 {
          tunnel: w227 -> [w235 w239]
          tunnel: [w238 w239] -> w226
          tunnel: w222 -> [w237 _]
          frame 1 {
            n99 = local read "Coords"() -> (w236:T1)
            n100 = Unbundle By Name(w235) -> ("Double Click"=w233:bool)
            n101 = Equal?(x=w237, y=w236) -> (x = y?=w234:bool)
            n102 = Select(t=FALSE, s=w234, f=w233) -> (s? t:f=w231:bool)
            n103 = Bundle By Name(cluster=w235, "Double Click"=w231) -> (w238:cluster{"Double Click":bool, "Menu Key":bool})
          }
          frame 0, Default {
          }
        }
        n104 = event-data("Button"=w223, "Mods"=w226, "PlatMods"=w225, "Discard?"=FALSE) -> ()  [unwired: 1 in, 1 out]
      }
    }
    n105 = control-ref of="Colormap"() -> (w17:refnum<vi>)
    n106 = control-ref of="This VI"() -> (w12:refnum<vi>)
    n107 = Unbundle By Name(w19) -> ("Refnum"=w18:refnum<vi>)
    n108 = call <vilib>:"svx_Colormap Exec Commands.vi"("Container ref"=w18, "This VI"=w12, "Colormap ref"=w17, "Events"=w16, "State in"=w9, "Data in"=w20) -> ("State out"=w8:T3)  [unwired: 5 in]
  }
  "Display State Out" <- w4
  "Data Out" <- w2
  "Action" <- w3
